vi "Page_Info_Write.vi"(6 "ctlReferences":T1, 8 "error in (no error)":errorcluster, 11 "Installer.lvclass":refnum<class "Installer.lvclass">) -> (0 "error out":errorcluster, 3 "Installer.lvclass":refnum<class "Installer.lvclass">)   [LabVIEW 2020, in "Installer.lvclass"]
uses:
  <vilib>/AppBuilder/IB_Classes/Installer/Installer.lvclass
  <resource>/Framework/Providers/Builds/Installer/Pages/controls/IB_UI_Page_Info_References.ctl
  <vilib>/AppBuilder/IB_Classes/Installer/Installer.lvclass/Installer.ctl
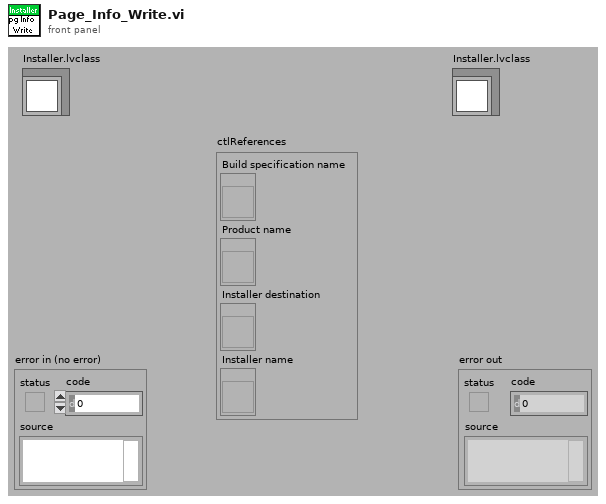
[diagram p1: front panel]
types:
  T1 = typedef "IB_UI_Page_Info_References.ctl" = cluster{"Build specification name":refnum<vi>, "Product name":refnum<vi>, "Installer destination":refnum<vi>, "Installer name":refnum<vi>}
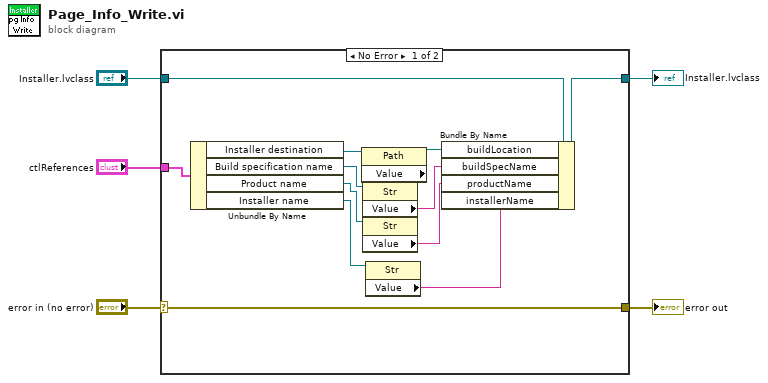
[diagram p0: block diagram]
diagram:
  n1 = case shown="No Error" "error in (no error)" {
    selector: "error in (no error)" -> [w10 w19]
    tunnel: [w10 w19] -> w4
    tunnel: "ctlReferences" -> [w17 _]
    tunnel: "Installer.lvclass" -> [w9 w18]
    tunnel: [w8 w18] -> w1
    frame No Error {
      n2 = Unbundle By Name(w17) -> ("Installer destination"=w12:refnum<vi>, "Build specification name"=w16:refnum<vi>, "Product name"=w15:refnum<vi>, "Installer name"=w7:refnum<vi>)
      n3 = property class="Path"(reference=w12) -> ("Value"=w11:path)  [unwired: 1 in, 2 out]
      n4 = property class="Str"(reference=w16) -> ("Value"=w13:string)  [unwired: 1 in, 2 out]
      n5 = property class="Str"(reference=w15) -> ("Value"=w14:string)  [unwired: 1 in, 2 out]
      n6 = property class="Str"(reference=w7) -> ("Value"=w6:string)  [unwired: 1 in, 2 out]
      n7 = Bundle By Name(cluster=w9, "buildLocation"=w11, "buildSpecName"=w13, "productName"=w14, "installerName"=w6) -> (w8:refnum<class "Installer.lvclass">)
    }
    frame Error {
    }
  }
  "error out" <- w4
  "Installer.lvclass" <- w1
